vi "Serial tester.vi"() -> ()   [LabVIEW 2019]
uses:
  Program Files (x86)/National Instruments/LabVIEW 2019/examples/Instrument IO/Serial/support/Serial - Settings.ctl
  <vilib>/Instr/_visa.llb/VISA Configure Serial Port (Instr).vi
panel:
  in  "wait":u32
  out "status byte":u16
  out "return count":u32
  out "error out":errorcluster
  out "VISA resource name out":refnum<visa-resource-name>
  in  "reference":refnum<visa-resource-name>
  out "read buffer":string
  in  "error in (no error)":errorcluster
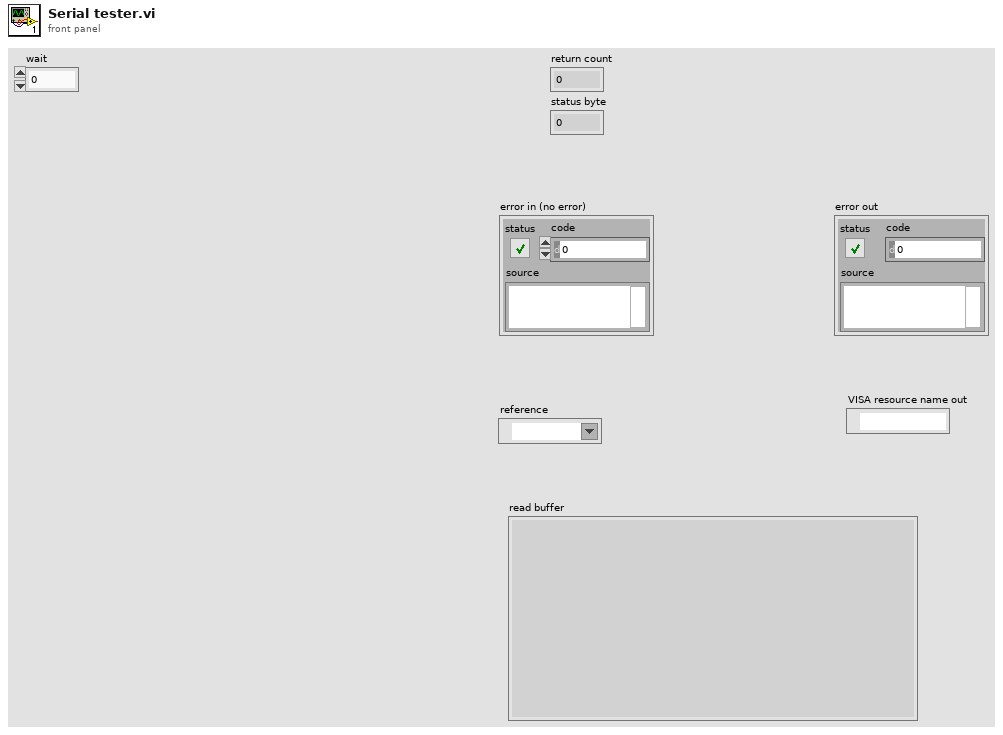
[diagram p1: front panel]
types:
  T1 = typedef "Serial - Settings.ctl" = cluster{"baud rate":u32, "data bits":u16, "parity":enum16{"None", "Odd", "Even", "Mark", "Space"}, "stop bits":u16, "flow control":u16}
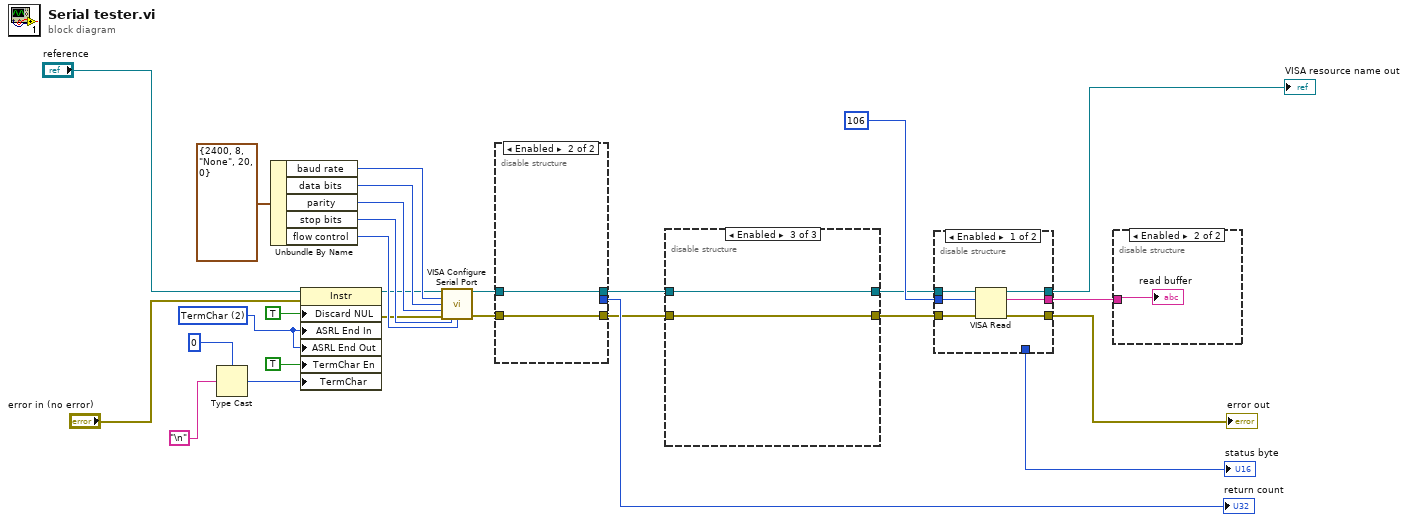
[diagram p0: block diagram]
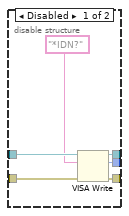
[diagram p2: hidden frame]
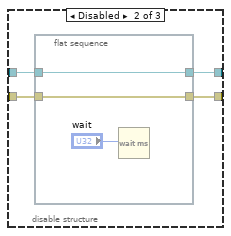
[diagram p4: hidden frame]
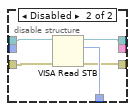
[diagram p5: hidden frame]
diagram:
  w23 = u16 2 items=["None", "Last Bit", "TermChar"] ("Serial Settings:End Mode for Reads")
  n1 = Type Cast(type=0, x="\n") -> (*(type *) &x=w21:i32)
  n2 = Unbundle By Name(T1 {"baud rate"=2400, "data bits"=8, "parity"=enum."None", "stop bits"=20, "flow control"=0} ("input cluster")) -> ("baud rate"=w28:u32, "data bits"=w27:u16, "parity"=w26:enum16{"None", "Odd", "Even", "Mark", "Space"}, "stop bits"=w25:u16, "flow control"=w24:u16)
  n3 = property class="Instr"(reference="reference", error in="error in (no error)", "Discard NUL"=TRUE ("Serial Settings:Discard NUL Characters"), "ASRL End In"=w23, "ASRL End Out"=w23, "TermChar En"=TRUE ("Message Based Settings:Termination Character Enable"), "TermChar"=w21) -> (reference out=w19:refnum<visa-resource-name>, error out=w20:errorcluster)
  n4 = call-poly "VISA Configure Serial Port"("VISA resource name"=w19, "baud rate (9600)"=w28, "data bits (8)"=w27, "parity (0:none)"=w26, "error in (no error)"=w20, "stop bits (10: 1 bit)"=w25, "flow control (0:none)"=w24) -> ("VISA resource name out"=w15:refnum<visa-resource-name>, "error out"=w18:errorcluster)  [unwired: 7 in]
  n5 = disable-structure shown="Enabled" {
    disable-tunnel: w18 -> [w34 w35]
    disable-tunnel: w15 -> [w33 w36]
    disable-tunnel: [w31 _] -> w7
    disable-tunnel: [w30 w36] -> w5
    disable-tunnel: [w29 w35] -> w3
    frame Disabled {
      n6 = VISA Write(VISA resource name=w33, write buffer="*IDN?" ("Command"), error in (no error)=w34) -> (VISA resource name out=w30:refnum<visa-resource-name>, return count=w31:u32, error out=w29:errorcluster)
    }
    frame Enabled {
    }
  }
  "return count" <- w7
  n7 = disable-structure shown="Enabled" {
    disable-tunnel: w5 -> [w38 w42 w47]
    disable-tunnel: [w38 w41 w47] -> w4
    disable-tunnel: [w37 w39 w46] -> w2
    disable-tunnel: w3 -> [w37 w40 w46]
    frame Disabled {
    }
    frame Disabled {
      n8 = flat-sequence {
        tunnel: w42 -> [w44]
        tunnel: [w44] -> w41
        tunnel: w40 -> [w43]
        tunnel: [w43] -> w39
        frame #0 {
          n9 = Wait (ms)(milliseconds to wait="wait") -> ()  [unwired: 1 out]
        }
      }
    }
    frame Enabled {
    }
  }
  n10 = disable-structure shown="Enabled" {
    disable-tunnel: w4 -> [w53 w58]
    disable-tunnel: w2 -> [w52 w57]
    disable-tunnel: u32 106 ("byte count") -> [w51 _]
    disable-tunnel: [w50 _] -> w12
    disable-tunnel: [w49 w55] -> w9
    disable-tunnel: [w48 w54] -> w8
    disable-tunnel: [_ w56] -> w6
    frame Enabled {
      n11 = VISA Read(VISA resource name=w53, byte count=w51, error in (no error)=w52) -> (VISA resource name out=w49:refnum<visa-resource-name>, read buffer=w50:string, error out=w48:errorcluster)  [unwired: 1 out]
    }
    frame Disabled {
      n12 = VISA Read STB(8:w57, 11:w58) -> (0:w54:errorcluster, 2:w56:u16, 3:w55:refnum<visa-resource-name>)
    }
  }
  "VISA resource name out" <- w9
  "error out" <- w8
  "status byte" <- w6
  n13 = disable-structure shown="Enabled" {
    disable-tunnel: w12 -> [_ w59]
    frame Disabled {
    }
    frame Enabled {
      "read buffer" <- w59
    }
  }
